vi "CT_VFModifyPiezoPuffTrig.vi"(1 "Form Index":i32=1, 2 "Ultra Fast Timing In":dbl[](array[slide])=[1100.0, 3200.0, 3254.0, 3290.0, 3100.0, 3080.0, 0.0, 3100.0] min=0.0 max=4000.0 step=2.0 scale=0.0..4000.0 scale format="%#_3f", 3 "Fake Form Index":i32=1, 5 "Puff Index":i32, 6 "Very Fast Timing In":dbl[](array[slide])=[1100.0, 3200.0, 3254.0, 3290.0, 3100.0, 3080.0, 0.0, 3100.0] min=0.0 max=4000.0 step=2.0 scale=0.0..4000.0 scale format="%#_3f") -> (0 "Very Fast Timing Out":dbl[](array[slide])=[1100.0, 3200.0, 3254.0, 3290.0, 3100.0, 3080.0, 0.0, 3100.0] min=0.0 max=4000.0 step=2.0 scale=0.0..4000.0 scale format="%#_3f")   [LabVIEW 2016]
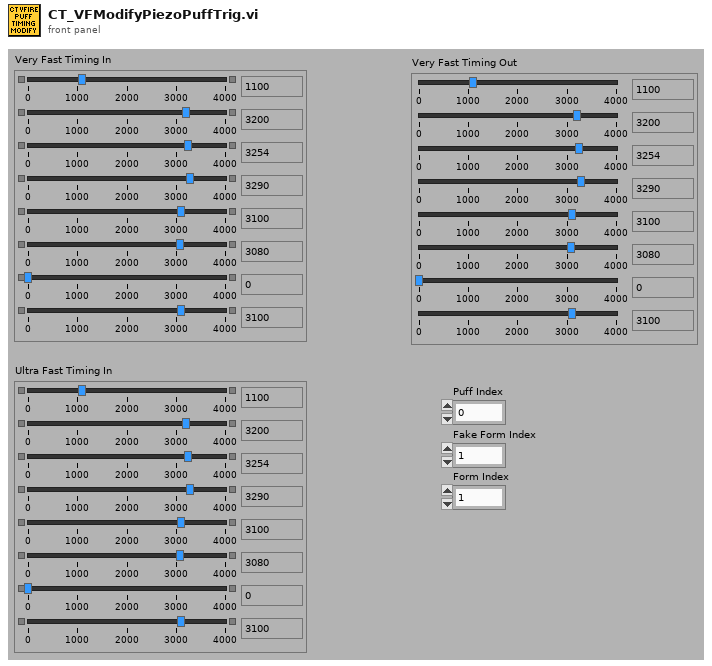
[diagram p1: front panel]
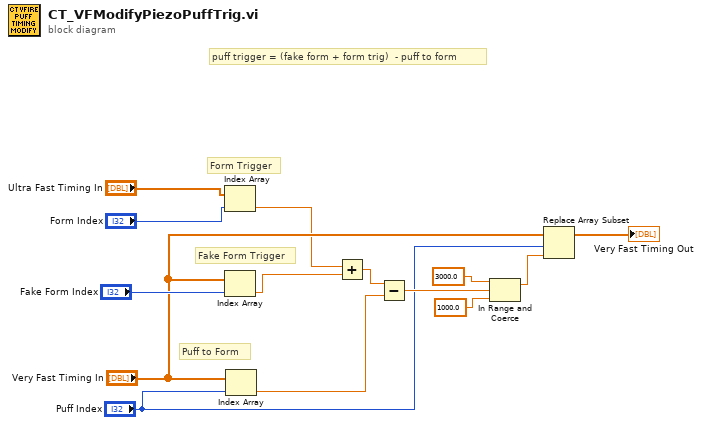
[diagram p0: block diagram]
diagram:
  # "Form Trigger"
  # "puff trigger = (fake form + form trig)  - puff to form"
  # "Fake Form Trigger"
  # "Puff to Form"
  n1 = Index Array(array="Ultra Fast Timing In", index="Form Index") -> (element=w4:dbl)
  n2 = Index Array(array="Very Fast Timing In", index="Fake Form Index") -> (element=w3:dbl)
  n3 = Index Array(array="Very Fast Timing In", index="Puff Index") -> (element=w1:dbl)
  n4 = Add(x=w4, y=w3) -> (x+y=w2:dbl)
  n5 = Subtract(x=w2, y=w1) -> (x-y=w11:dbl)
  n6 = In Range and Coerce(upper limit=3000.0, x=w11, lower limit=1000.0) -> (coerced(x)=w10:dbl)  [unwired: 1 out]
  n7 = Replace Array Subset(array="Very Fast Timing In", new element=w10, index="Puff Index") -> (→"Very Fast Timing Out":dbl[])
